vi "SetDigitalPWM.vi"(0 "Connexion réseau UDP en entrée":refnum<k16>, 1 "Pin":u8, 2 "entrée d'erreur (pas d'erreur)":errorcluster, 3 "Adresse IP":u32, 4 "Value In":u8=1 caption="Value [0 - 255]", 5 "Port Distant":u16) -> (6 "Connexion réseau UDP en sortie":refnum<k16>, 7 "error out":errorcluster caption="sortie d'erreur", 8 "Return Value":u8)   [LabVIEW 2021]
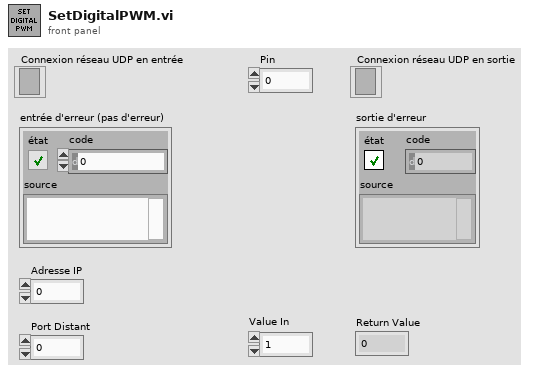
[diagram p1: front panel]
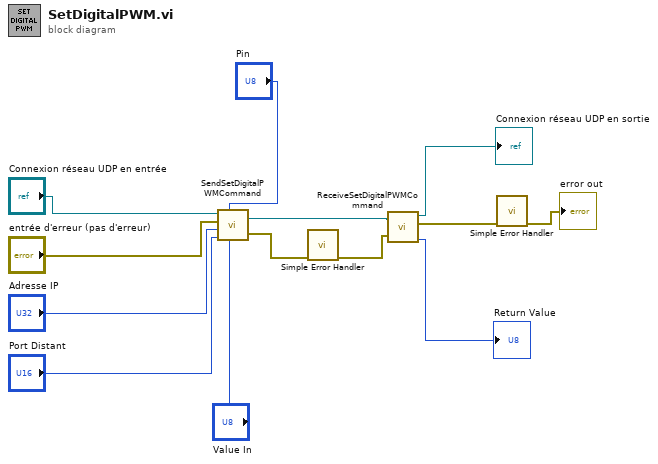
[diagram p0: block diagram]
diagram:
  n1 = call "SendSetDigitalPWMCommand.vi"(2:"Value In", 3:"Pin", "Port Distant"="Port Distant", "Addresse IP"="Adresse IP", "entrée d'erreur (pas d'erreur)"="entrée d'erreur (pas d'erreur)", "Connexion réseau UDP en entrée"="Connexion réseau UDP en entrée") -> ("sortie d'erreur"=w8:errorcluster, "Connexion réseau UDP en sortie"=w4:refnum<k16>)
  n2 = call <vilib>:"Simple Error Handler.vi"("error in (no error)"=w8) -> ("error out"=w5:errorcluster)  [unwired: 4 in, 4 out]
  n3 = call "ReceiveSetDigitalPWMCommand.vi"("Connexion réseau UDP en entrée"=w4, "entrée d'erreur (pas d'erreur)"=w5) -> ("Connexion réseau UDP en sortie"=→"Connexion réseau UDP en sortie":refnum<k16>, "sortie d'erreur"=w2:errorcluster, "Value"=→"Return Value":u8)  [unwired: 1 out]
  n4 = call <vilib>:"Simple Error Handler.vi"("error in (no error)"=w2) -> ("error out"=→"error out":errorcluster)  [unwired: 4 in, 4 out]
